vi "ClimbSimple.vi"() -> ()   [LabVIEW 2013]
uses:
  Robot Global Data.vi
  ClimbStatesSimple.ctl
  <vilib>/Rock Robotics/SystemInterfaces/DIO/FPGA_DIOChannel.ctl
  <vilib>/Rock Robotics/SystemInterfaces/Typedef/FPGA_TypedefDigitalModule.ctl
  <vilib>/Rock Robotics/WPI/DigitalInput/WPI_DigitalInputDevRef.ctl
panel:
  out "ResumeState":T1
  out "CommandState":T1
  in  "input cluster":T5={"ArmInOut"={"DevStatus"={"status"=FALSE, "code"=0, "source"=""}, "DIO Channel"=enum."Invalid", "Digital Module"=enum."Digital Module 1"}, "ArmMiddle"={"DevStatus"={"status"=FALSE, "code"=0, "source"=""}, "DIO Channel"=enum."Invalid", "Digital Module"=enum."Digital Module 1"}, "HooksOut"={"DevStatus"={"status"=FALSE, "code"=0, "source"=""}, "DIO Channel"=enum."Invalid", "Digital Module"=enum."Digital Module 1"}, "HooksIn"={"DevStatus"={"status"=FALSE, "code"=0, "source"=""}, "DIO Channel"=enum."Invalid", "Digital Module"=enum."Digital Module 1"}, "HooksMiddle"={"DevStatus"={"status"=FALSE, "code"=0, "source"=""}, "DIO Channel"=enum."Invalid", "Digital Module"=enum."Digital Module 1"}, "Shooter"={"DevStatus"={"status"=FALSE, "code"=0, "source"=""}, "DIO Channel"=enum."Invalid", "Digital Module"=enum."Digital Module 1"}}
  out "ArmInOut":bool
  out "ArmMiddle":bool
  out "HooksOut":bool
  out "HooksIn":bool
  out "HooksMiddle":bool
  out "Shooter":bool
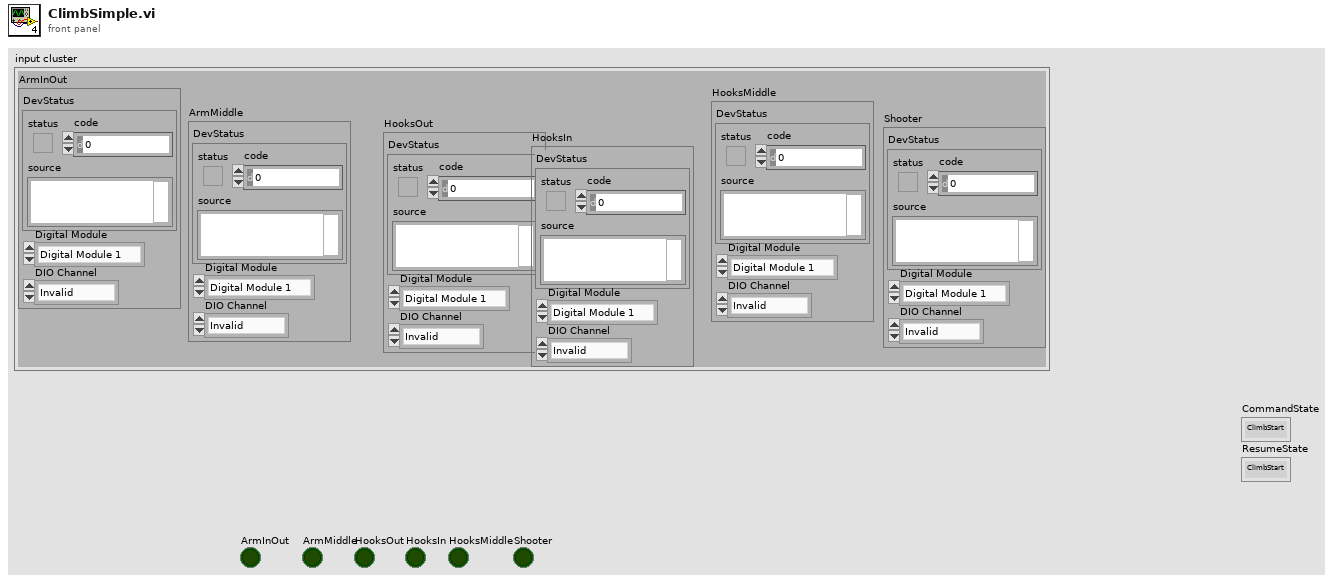
[diagram p1: front panel]
types:
  T1 = typedef "ClimbStatesSimple.ctl" = enum16{"ClimbStart", "ArmExtends", "Rachet re-engage", "Arm 60deg", "PullRobot", "Pause"}
  T2 = typedef "WPI_DigitalInputDevRef.ctl" = cluster{"DevStatus":errorcluster, "DIO Channel":T3, "Digital Module":T4}
  T3 = typedef "FPGA_DIOChannel.ctl" = enum8{"DIO 1", "DIO 2", "DIO 3", "DIO 4", "DIO 5", "DIO 6", "DIO 7", "DIO 8", "DIO 9", "DIO 10", "DIO 11", "DIO 12", "DIO 13", "DIO 14", "Invalid"}
  T4 = typedef "FPGA_TypedefDigitalModule.ctl" = enum16{"Digital Module 1", "Digital Module 2"}
  T5 = cluster{"ArmInOut":T2, "ArmMiddle":T2, "HooksOut":T2, "HooksIn":T2, "HooksMiddle":T2, "Shooter":T2}
  T6 = typedef "LoopDisable.ctl" = cluster{"Climb.vi":bool, "LauncherAngle.vi":bool, "Launcher.vi":bool, "ArmControl.vi":bool, "WinchMotor.vi":bool, "ReadDriveEncoder.vi":bool}
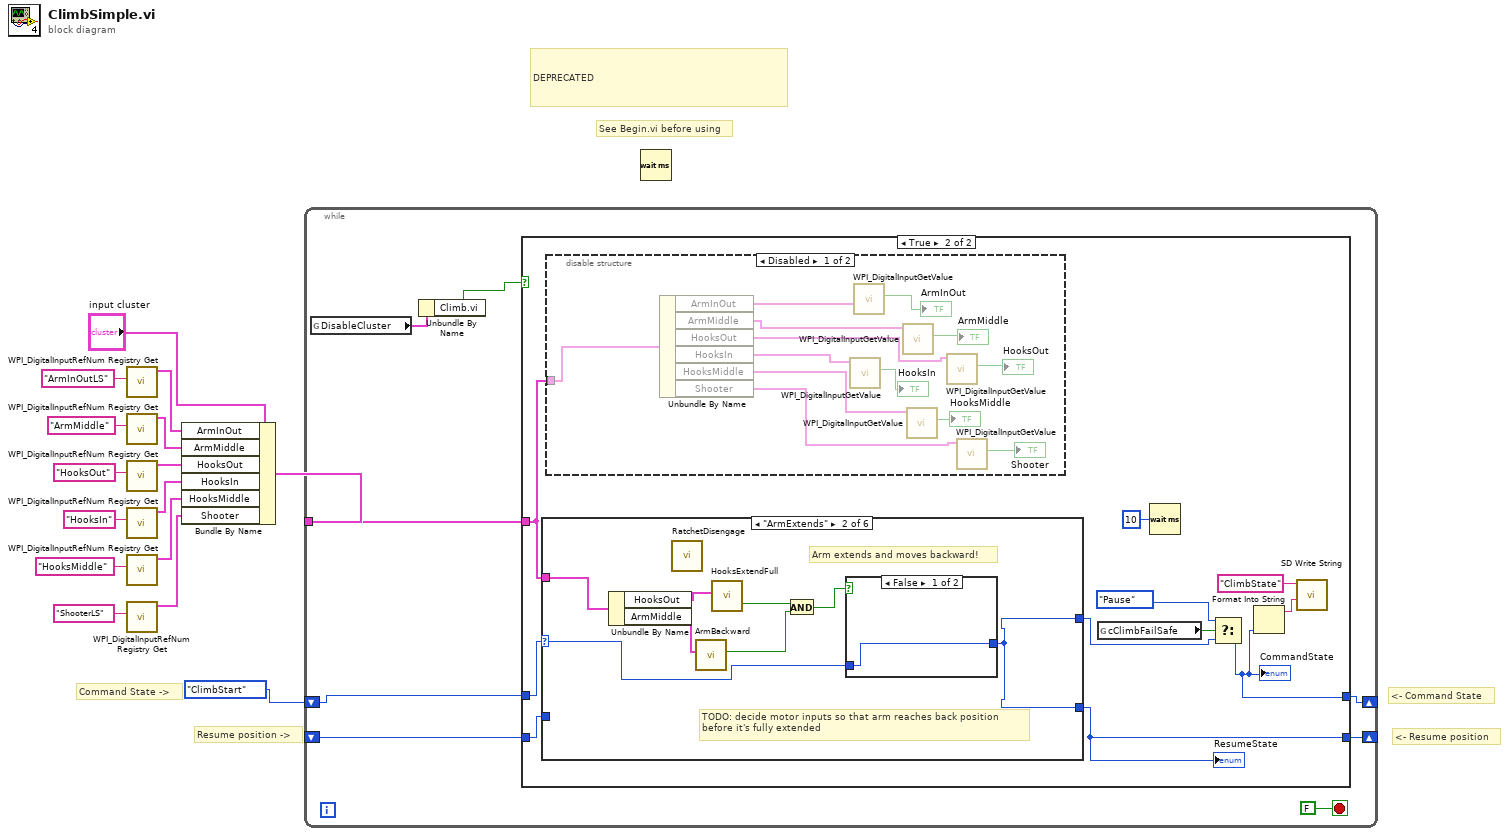
[diagram p0: block diagram]
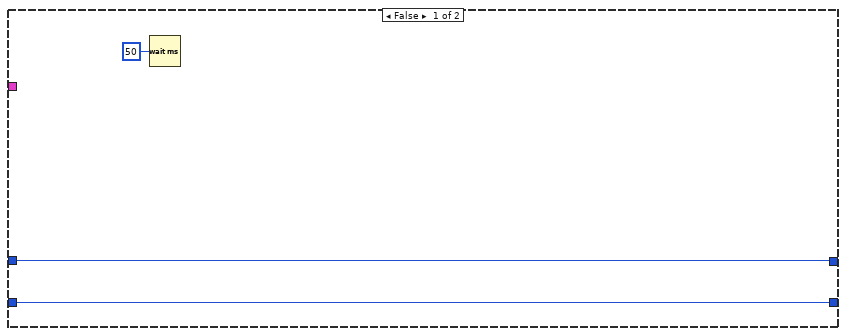
[diagram p2: hidden frame]
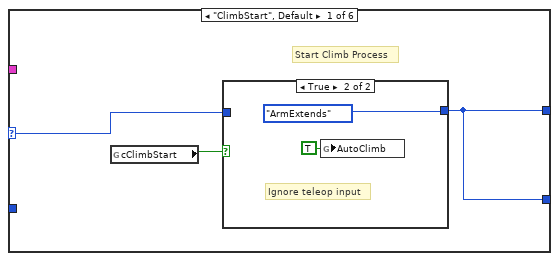
[diagram p3: hidden frame]
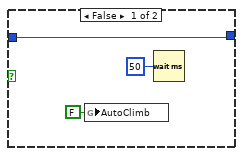
[diagram p4: hidden frame]
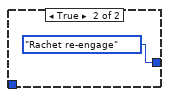
[diagram p5: hidden frame]
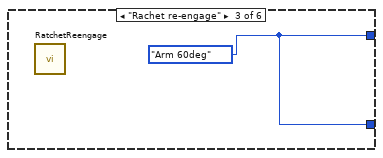
[diagram p6: hidden frame]
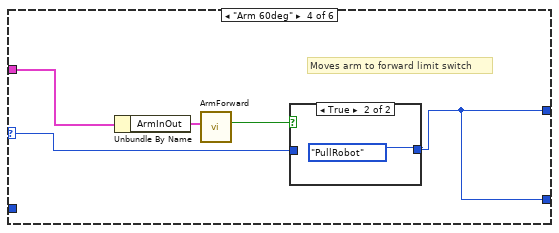
[diagram p7: hidden frame]
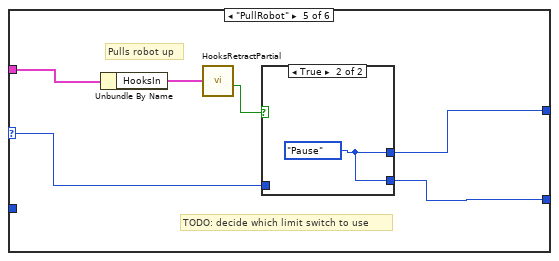
[diagram p9: hidden frame]
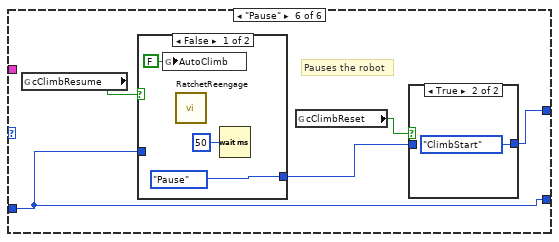
[diagram p11: hidden frame]
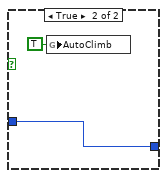
[diagram p13: hidden frame]
diagram:
  # "See Begin.vi before using"
  # "DEPRECATED"
  # "Resume position ->"
  # "Command State ->"
  # "<- Resume position"
  # "<- Command State"
  n1 = call <vilib>:"WPI_DigitalInputRefNum Registry Get.vi"("refnum name"="ArmInOutLS") -> ("DigitalInputDevRef"=w9:T2)  [unwired: 9 in, 1 out]
  n2 = call <vilib>:"WPI_DigitalInputRefNum Registry Get.vi"("refnum name"="ArmMiddle") -> ("DigitalInputDevRef"=w7:T2)  [unwired: 9 in, 1 out]
  n3 = call <vilib>:"WPI_DigitalInputRefNum Registry Get.vi"("refnum name"="HooksOut") -> ("DigitalInputDevRef"=w6:T2)  [unwired: 9 in, 1 out]
  n4 = call <vilib>:"WPI_DigitalInputRefNum Registry Get.vi"("refnum name"="HooksIn") -> ("DigitalInputDevRef"=w5:T2)  [unwired: 9 in, 1 out]
  n5 = call <vilib>:"WPI_DigitalInputRefNum Registry Get.vi"("refnum name"="HooksMiddle") -> ("DigitalInputDevRef"=w4:T2)  [unwired: 9 in, 1 out]
  n6 = call <vilib>:"WPI_DigitalInputRefNum Registry Get.vi"("refnum name"="ShooterLS") -> ("DigitalInputDevRef"=w3:T2)  [unwired: 9 in, 1 out]
  n7 = Bundle By Name(cluster="input cluster", "ArmInOut"=w9, "ArmMiddle"=w7, "HooksOut"=w6, "HooksIn"=w5, "HooksMiddle"=w4, "Shooter"=w3) -> (w2:T5)
  n8 = while {
    shift-right: [w21] -> _
    shift-left: _ -> [w22]
    tunnel: w2 -> [w20]
    shift-right: [w18] -> _
    shift-left: ClimbStatesSimple."ClimbStart" ("Enum") -> [w17]
    stop <- FALSE stop-if-true
    n9 = global read "Robot Global Data.vi" "DisableCluster"() -> (w19:T6)
    n10 = Unbundle By Name(w19) -> ("Climb.vi"=w16:bool)
    n11 = case shown="True" w16 {
      tunnel: w17 -> [w26 w32]
      tunnel: w22 -> [w25 w31]
      tunnel: [w25 w27] -> w21
      tunnel: [w26 w28] -> w18
      tunnel: w20 -> [_ w30]
      frame False {
        n12 = Wait (ms)(milliseconds to wait=u32 50) -> ()  [unwired: 1 out]
      }
      frame True {
        n13 = case shown="\"ArmExtends\"" w32 {
          selector: w32 -> [w39 w48 _ w59 w66 _]
          tunnel: w31 -> [_ _ _ _ _ w73]
          tunnel: w30 -> [_ w46 _ w58 w67 _]
          tunnel: [w38 w47 w56 w57 w64 w72] -> w29
          tunnel: [w38 w47 w56 w57 w65 w73] -> w27
          frame "ClimbStart", Default {
            # "Start Climb Process"
            n14 = global read "Robot Global Data.vi" "cClimbStart"() -> (w40:bool)
            n15 = case shown="True" w40 {
              tunnel: [w41 ClimbStatesSimple."ArmExtends" ("Enum")] -> w38
              tunnel: w39 -> [w41 _]
              frame False {
                n16 = global write "Robot Global Data.vi" "AutoClimb"(FALSE ("AutoClimb")) -> ()
                n17 = Wait (ms)(milliseconds to wait=u32 50) -> ()  [unwired: 1 out]
              }
              frame True {
                # "Ignore teleop input"
                n18 = global write "Robot Global Data.vi" "AutoClimb"(TRUE ("AutoClimb")) -> ()
              }
            }
          }
          frame "ArmExtends" {
            # "TODO: decide motor inputs so that arm reaches back position\nbefore it's fully extended"
            # "Arm extends and moves backward!"
            n19 = Unbundle By Name(w46) -> ("HooksOut"=w53:T2, "ArmMiddle"=w52:T2)
            n20 = call "RatchetDisengage.vi"() -> ()  [unwired: 12 in]
            n21 = call "ArmBackward.vi"("BackwardLimitSwitch"=w52) -> ("Done?"=w50:bool)  [unwired: 10 in]
            n22 = call "HooksExtendFull.vi"("HooksOutLimitSwitch"=w53) -> ("Done?"=w51:bool)  [unwired: 10 in]
            n23 = And(x=w51, y=w50) -> (x .and. y?=w49:bool)
            n24 = case shown="False" w49 {
              tunnel: w48 -> [w54 _]
              tunnel: [w54 ClimbStatesSimple."Rachet re-engage" ("Enum")] -> w47
              frame False {
              }
              frame True {
              }
            }
          }
          frame "Rachet re-engage" {
            w56 = ClimbStatesSimple."Arm 60deg" ("Enum")
            n25 = call "RatchetReengage.vi"() -> ()  [unwired: 12 in]
          }
          frame "Arm 60deg" {
            # "Moves arm to forward limit switch"
            n26 = Unbundle By Name(w58) -> ("ArmInOut"=w61:T2)
            n27 = call "ArmForward.vi"("ForwardLimitSwitch"=w61) -> ("Done?"=w60:bool)  [unwired: 10 in]
            n28 = case shown="True" w60 {
              tunnel: w59 -> [w62 _]
              tunnel: [w62 ClimbStatesSimple."PullRobot" ("Enum")] -> w57
              frame False {
              }
              frame True {
              }
            }
          }
          frame "PullRobot" {
            # "TODO: decide which limit switch to use"
            # "Pulls robot up"
            n29 = Unbundle By Name(w67) -> ("HooksIn"=w69:T2)
            n30 = call "HooksRetractPartial.vi"("HooksMiddleLimitSwitch"=w69) -> ("Done?"=w68:bool)  [unwired: 10 in]
            n31 = case shown="True" w68 {
              tunnel: w66 -> [w70 _]
              tunnel: [w70 w71] -> w65
              tunnel: [w70 w71] -> w64
              frame False {
              }
              frame True {
                w71 = ClimbStatesSimple."Pause" ("Enum")
              }
            }
          }
          frame "Pause" {
            # "Pauses the robot"
            n32 = global read "Robot Global Data.vi" "cClimbResume"() -> (w76:bool)
            n33 = case shown="False" w76 {
              tunnel: w73 -> [_ w83]
              tunnel: [ClimbStatesSimple."Pause" ("Enum") w83] -> w74
              frame False {
                n34 = global write "Robot Global Data.vi" "AutoClimb"(FALSE ("AutoClimb")) -> ()
                n35 = call "RatchetReengage.vi"() -> ()  [unwired: 12 in]
                n36 = Wait (ms)(milliseconds to wait=u32 50) -> ()  [unwired: 1 out]
              }
              frame True {
                n37 = global write "Robot Global Data.vi" "AutoClimb"(TRUE ("AutoClimb")) -> ()
              }
            }
            n38 = global read "Robot Global Data.vi" "cClimbReset"() -> (w75:bool)
            n39 = case shown="True" w75 {
              tunnel: [w77 ClimbStatesSimple."ClimbStart" ("Enum")] -> w72
              tunnel: w74 -> [w77 _]
              frame False {
              }
              frame True {
              }
            }
          }
        }
        "ResumeState" <- w27
        n40 = disable-structure shown="Disabled" {
          disable-tunnel: w30 -> [w96 _]
          frame Disabled {
            n41 = Unbundle By Name(w96) -> ("ArmInOut"=w95:T2, "ArmMiddle"=w93:T2, "HooksOut"=w91:T2, "HooksIn"=w89:T2, "HooksMiddle"=w87:T2, "Shooter"=w85:T2)
            n42 = call <vilib>:"WPI_DigitalInputGetValue.vi"("DigitalInputDevRef"=w89) -> ("Value"=→"HooksIn":bool)  [unwired: 8 in, 2 out]
            n43 = call <vilib>:"WPI_DigitalInputGetValue.vi"("DigitalInputDevRef"=w95) -> ("Value"=→"ArmInOut":bool)  [unwired: 8 in, 2 out]
            n44 = call <vilib>:"WPI_DigitalInputGetValue.vi"("DigitalInputDevRef"=w93) -> ("Value"=→"ArmMiddle":bool)  [unwired: 8 in, 2 out]
            n45 = call <vilib>:"WPI_DigitalInputGetValue.vi"("DigitalInputDevRef"=w87) -> ("Value"=→"HooksMiddle":bool)  [unwired: 8 in, 2 out]
            n46 = call <vilib>:"WPI_DigitalInputGetValue.vi"("DigitalInputDevRef"=w91) -> ("Value"=→"HooksOut":bool)  [unwired: 8 in, 2 out]
            n47 = call <vilib>:"WPI_DigitalInputGetValue.vi"("DigitalInputDevRef"=w85) -> ("Value"=→"Shooter":bool)  [unwired: 8 in, 2 out]
          }
          frame Enabled {
          }
        }
        n48 = global read "Robot Global Data.vi" "cClimbFailSafe"() -> (w37:bool)
        n49 = Wait (ms)(milliseconds to wait=u32 10) -> ()  [unwired: 1 out]
        n50 = Select(t=ClimbStatesSimple."Pause" ("Enum"), s=w37, f=w29) -> (s? t:f=w28:T1)
        "CommandState" <- w28
        n51 = Format Into String(w28) -> (resulting string=w35:string)  [unwired: 3 in, 1 out]
        n52 = call <vilib>:"SD Write String.vi"("String"=w35, "Name"="ClimbState") -> ()  [unwired: 8 in, 2 out]
      }
    }
  }
  n53 = Wait (ms)() -> ()  [unwired: 1 in, 1 out]
